vi "Parse Get Topic Rule JSON.vi"(11 "Body":string) -> (3 "Topic Rule":T1)   [LabVIEW 2015, in "NI_AWS_IoT.lvlib"]
uses:
  NI_AWS_IoT.lvlib
  Topic Rule.ctl
  CloudWatch Alarm.ctl
  CloudWatch Metric.ctl
  DynamoDB.ctl
  DynamoDBv2.ctl
  Elasticsearch.ctl
  Firehose.ctl
  Kinesis.ctl
  Lambda.ctl
  Republish.ctl
  S3.ctl
  SNS.ctl
  SQS.ctl
  JSON Parsing/NI_JSON Parsing.lvlib
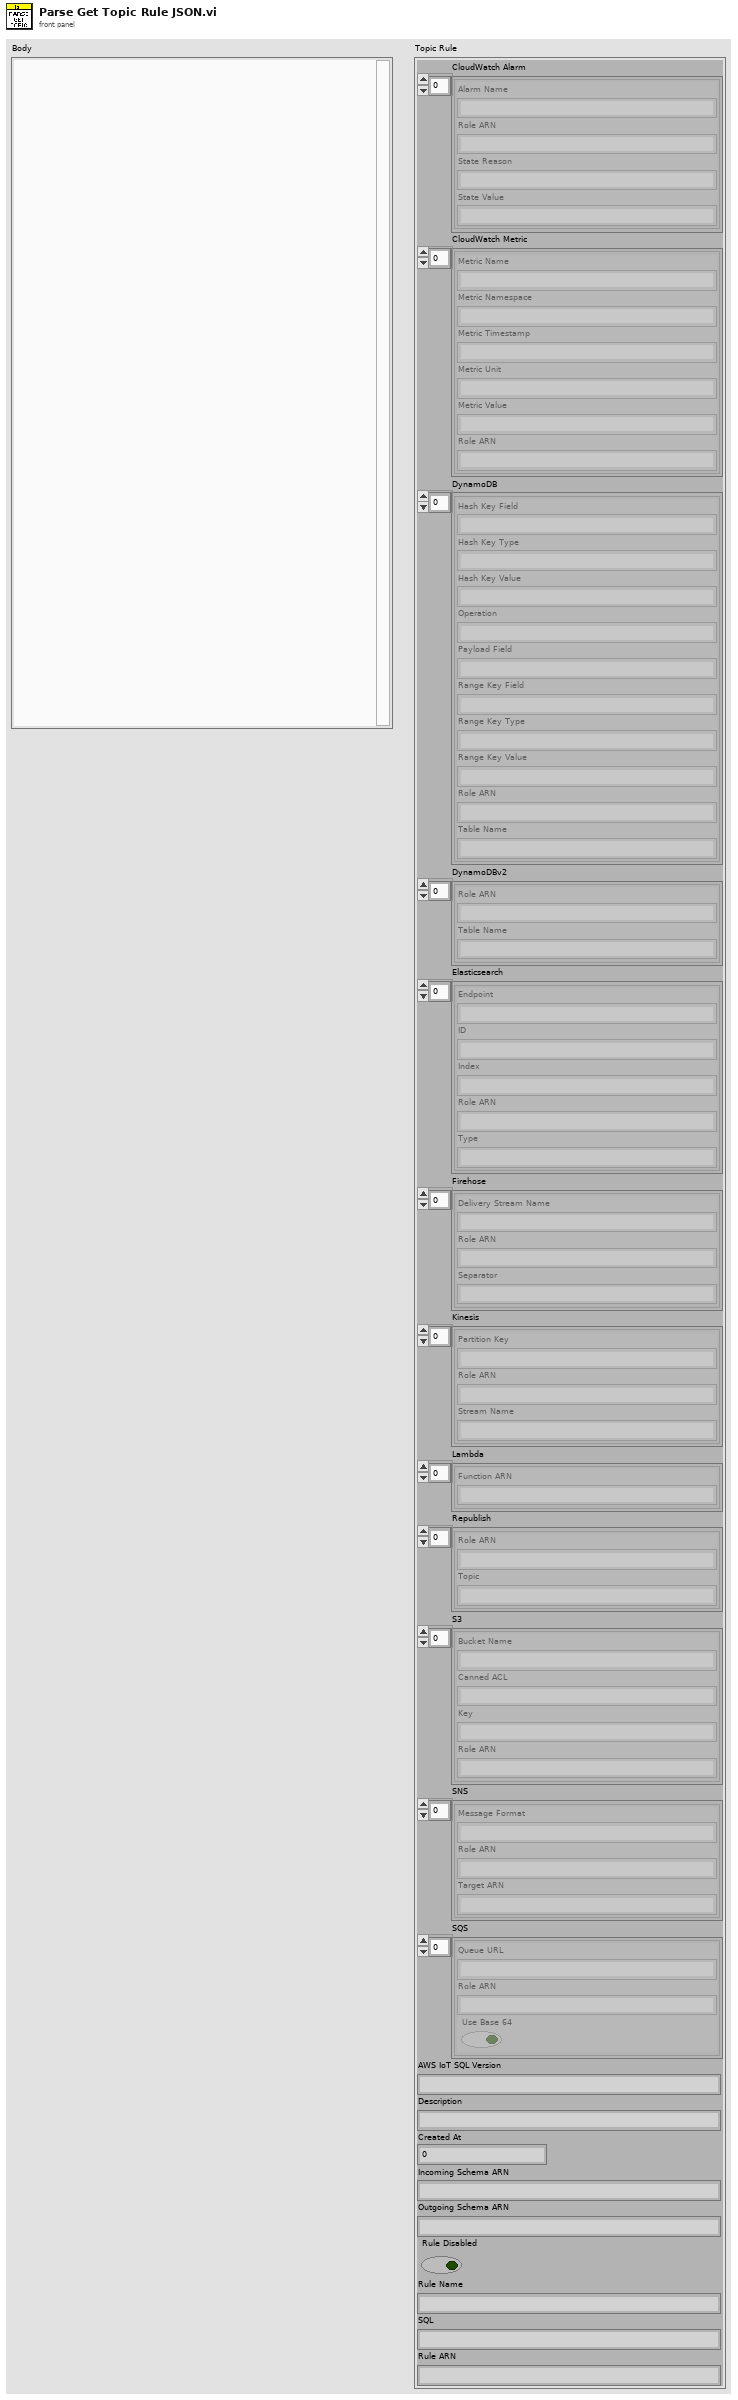
[diagram p1: front panel]
types:
  T1 = typedef "NI_AWS_IoT.lvlib/Topic Rule.ctl" = cluster{"CloudWatch Alarm":T2[], "CloudWatch Metric":T3[], "DynamoDB":T4[], "DynamoDBv2":T5[], "Elasticsearch":T6[], "Firehose":T7[], "Kinesis":T8[], "Lambda":T9[], "Republish":T10[], "S3":T11[], "SNS":T12[], "SQS":T13[], "AWS IoT SQL Version":string, "Description":string, "Created At":u64, "Incoming Schema ARN":string, "Outgoing Schema ARN":string, "Rule Disabled":bool, "Rule Name":string, "SQL":string, "Rule ARN":string}
  T2 = typedef "NI_AWS_IoT.lvlib/CloudWatch Alarm.ctl" = cluster{"Alarm Name":string, "Role ARN":string, "State Reason":string, "State Value":string}
  T3 = typedef "NI_AWS_IoT.lvlib/CloudWatch Metric.ctl" = cluster{"Metric Name":string, "Metric Namespace":string, "Metric Timestamp":string, "Metric Unit":string, "Metric Value":string, "Role ARN":string}
  T4 = typedef "NI_AWS_IoT.lvlib/DynamoDB.ctl" = cluster{"Hash Key Field":string, "Hash Key Type":string, "Hash Key Value":string, "Operation":string, "Payload Field":string, "Range Key Field":string, "Range Key Type":string, "Range Key Value":string, "Role ARN":string, "Table Name":string}
  T5 = typedef "NI_AWS_IoT.lvlib/DynamoDBv2.ctl" = cluster{"Role ARN":string, "Table Name":string}
  T6 = typedef "NI_AWS_IoT.lvlib/Elasticsearch.ctl" = cluster{"Endpoint":string, "ID":string, "Index":string, "Role ARN":string, "Type":string}
  T7 = typedef "NI_AWS_IoT.lvlib/Firehose.ctl" = cluster{"Delivery Stream Name":string, "Role ARN":string, "Separator":string}
  T8 = typedef "NI_AWS_IoT.lvlib/Kinesis.ctl" = cluster{"Partition Key":string, "Role ARN":string, "Stream Name":string}
  T9 = typedef "NI_AWS_IoT.lvlib/Lambda.ctl" = cluster{"Function ARN":string}
  T10 = typedef "NI_AWS_IoT.lvlib/Republish.ctl" = cluster{"Role ARN":string, "Topic":string}
  T11 = typedef "NI_AWS_IoT.lvlib/S3.ctl" = cluster{"Bucket Name":string, "Canned ACL":string, "Key":string, "Role ARN":string}
  T12 = typedef "NI_AWS_IoT.lvlib/SNS.ctl" = cluster{"Message Format":string, "Role ARN":string, "Target ARN":string}
  T13 = typedef "NI_AWS_IoT.lvlib/SQS.ctl" = cluster{"Queue URL":string, "Role ARN":string, "Use Base 64":bool}
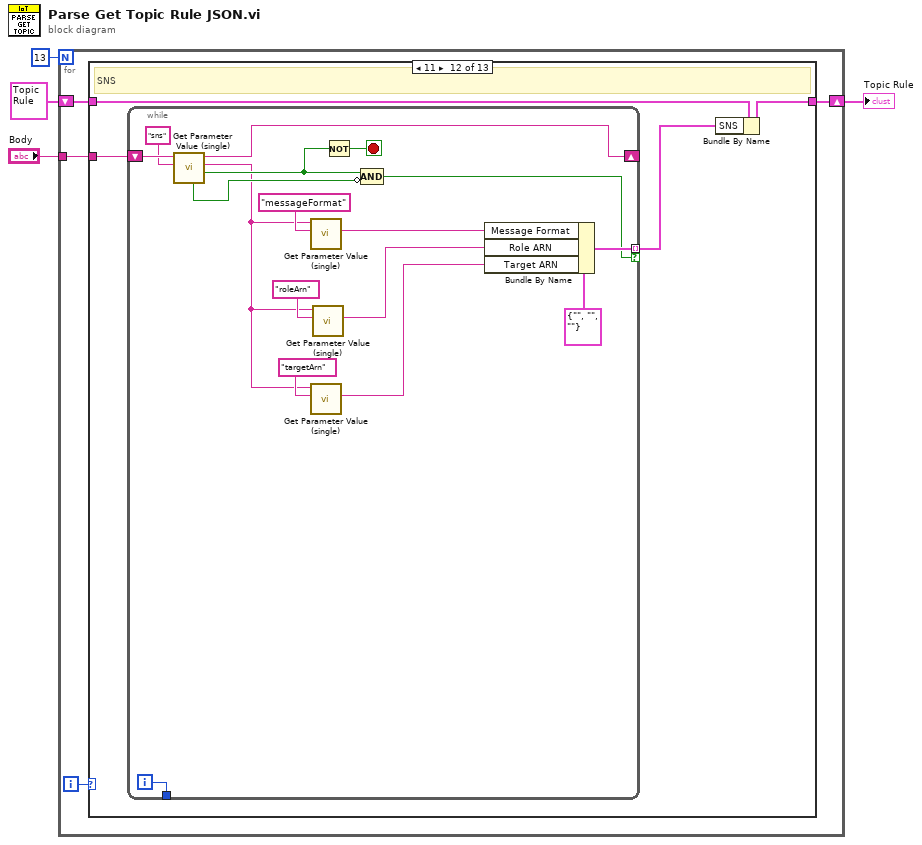
[diagram p0: block diagram]
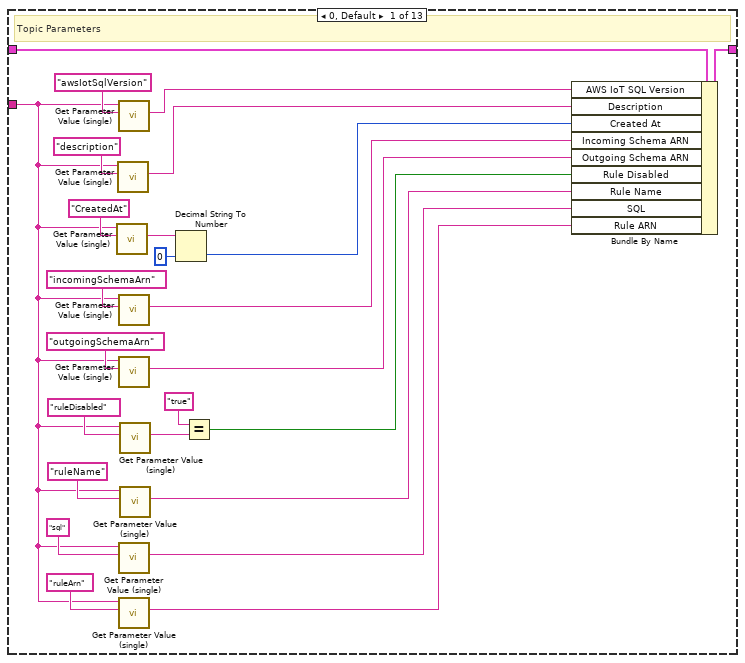
[diagram p2: hidden frame]
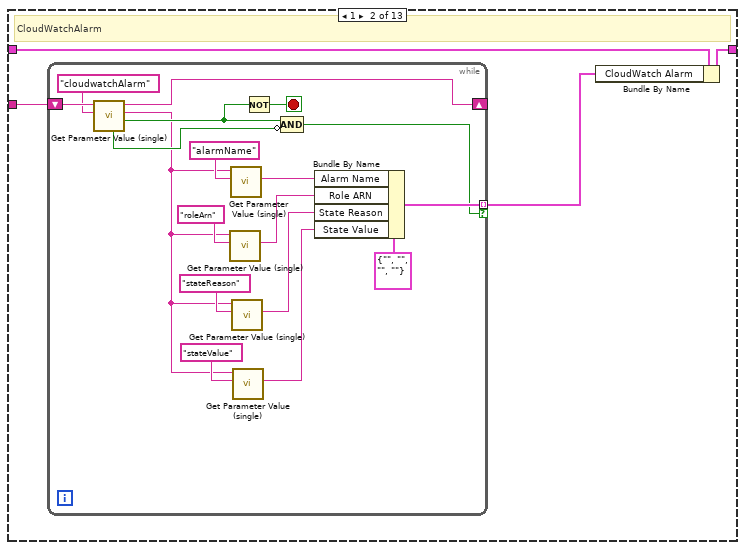
[diagram p3: hidden frame]
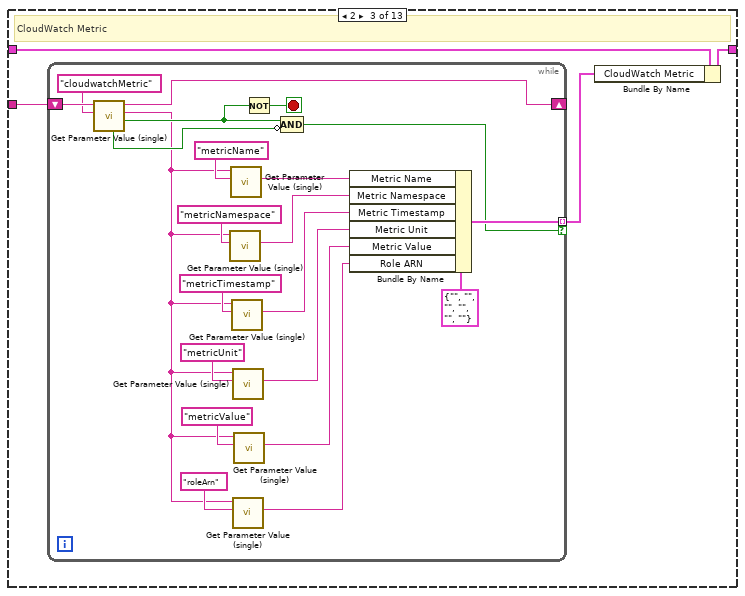
[diagram p4: hidden frame]
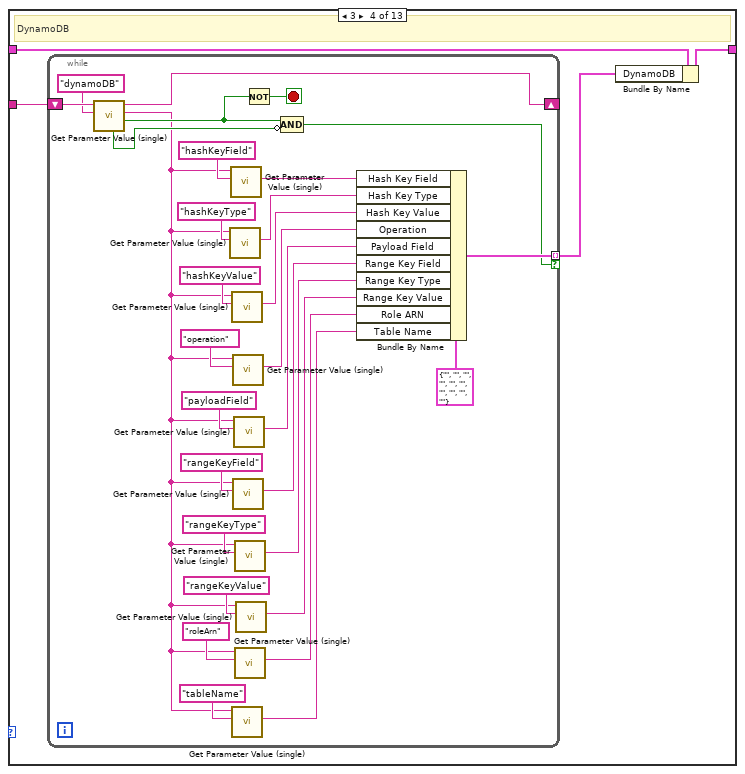
[diagram p5: hidden frame]
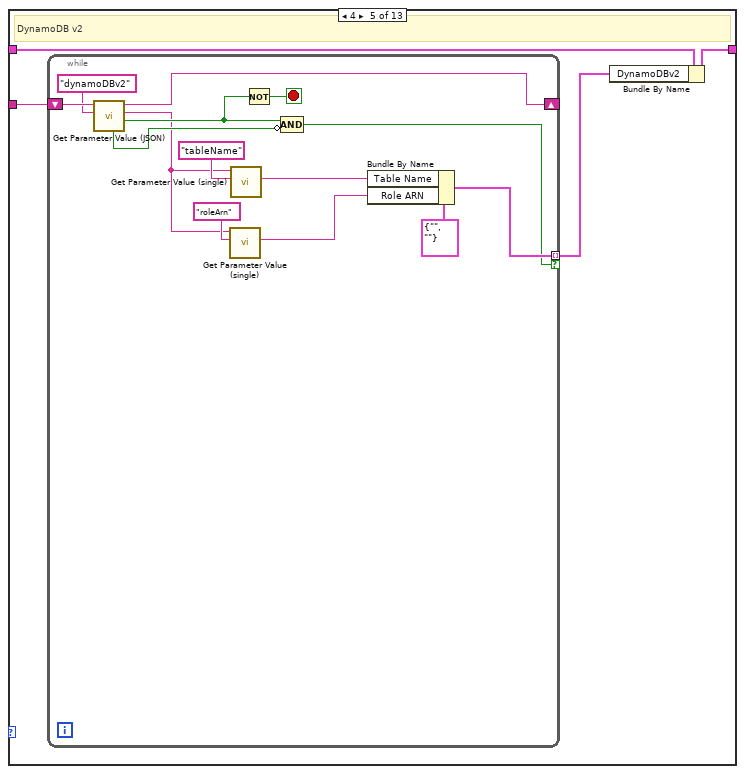
[diagram p6: hidden frame]
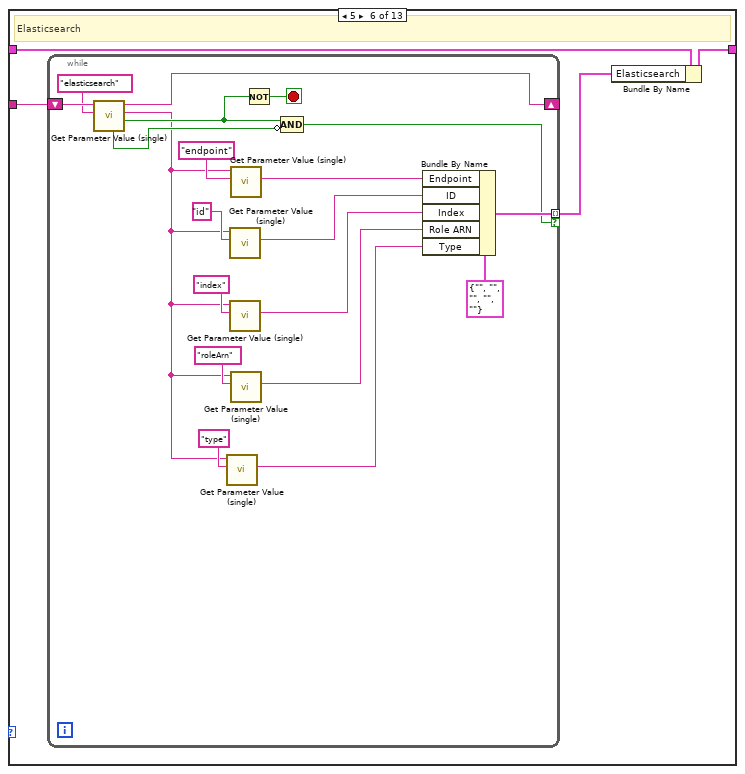
[diagram p7: hidden frame]
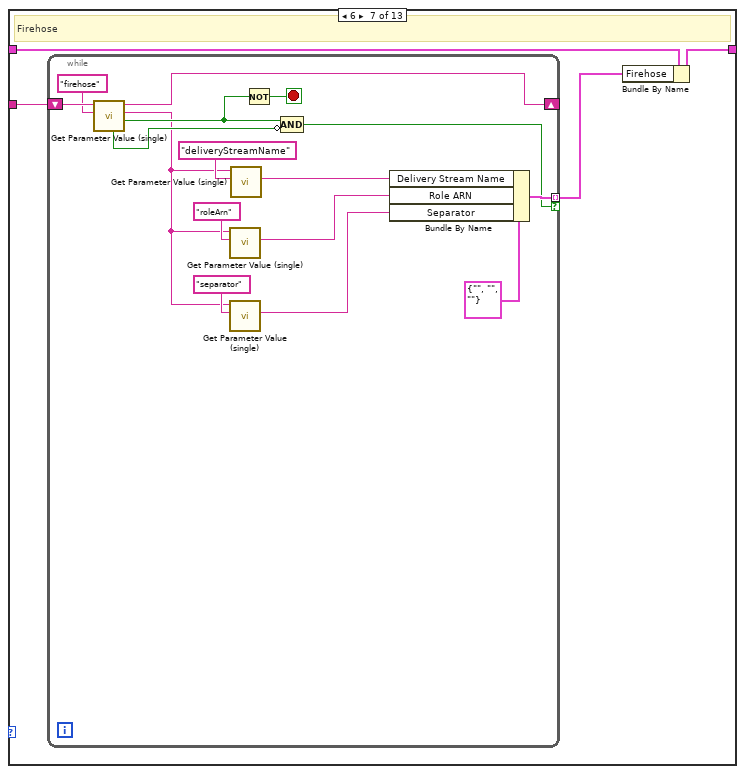
[diagram p8: hidden frame]
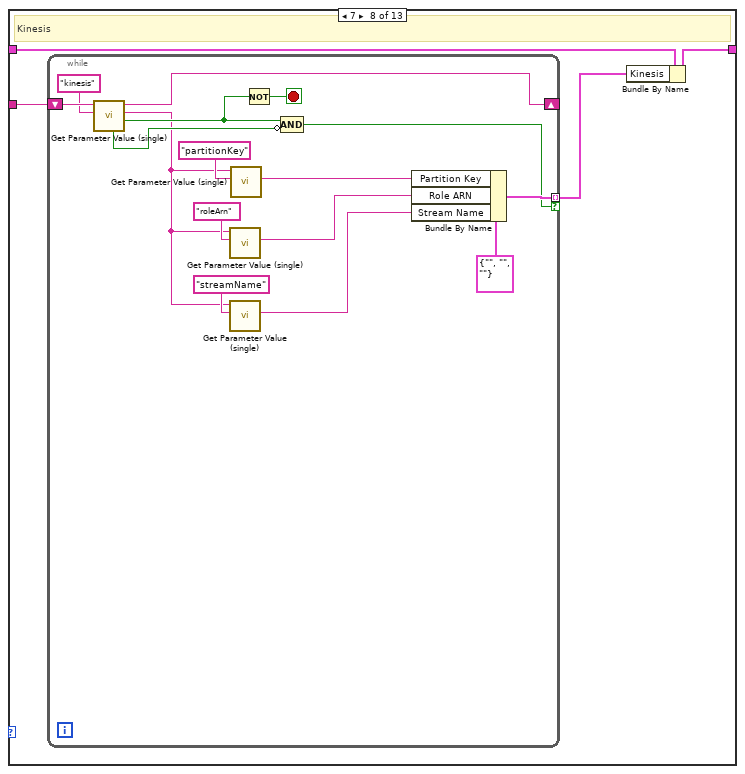
[diagram p9: hidden frame]
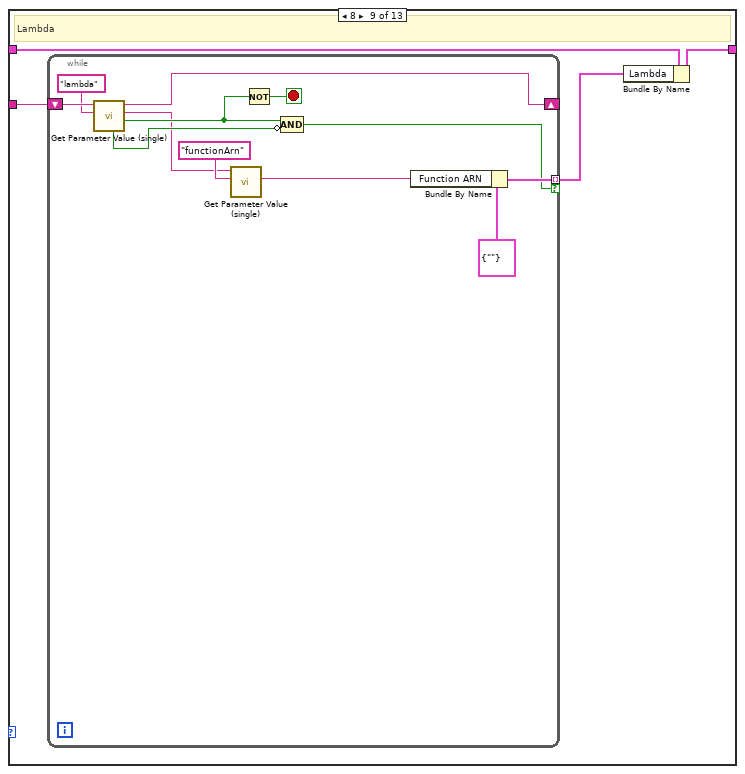
[diagram p10: hidden frame]
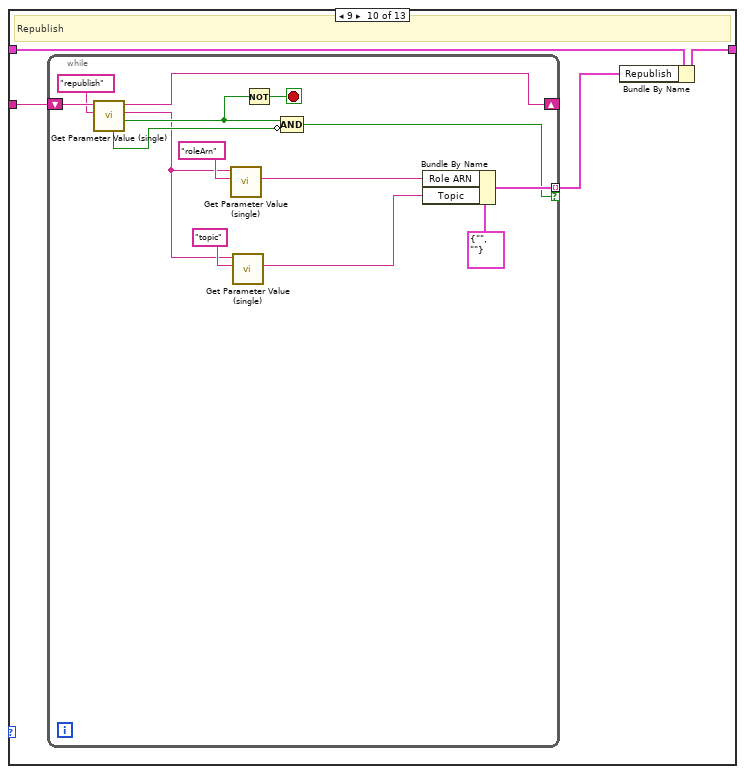
[diagram p11: hidden frame]
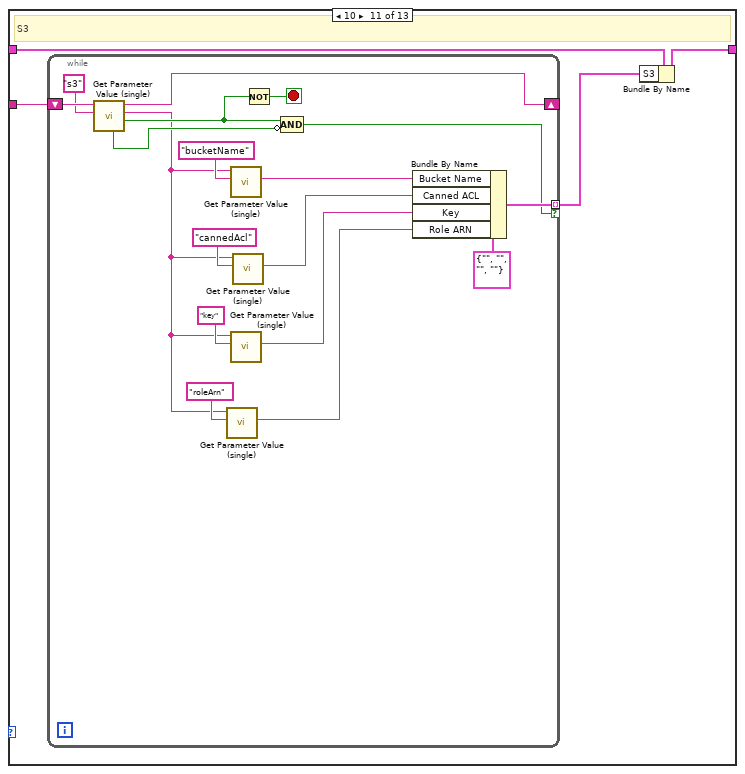
[diagram p12: hidden frame]
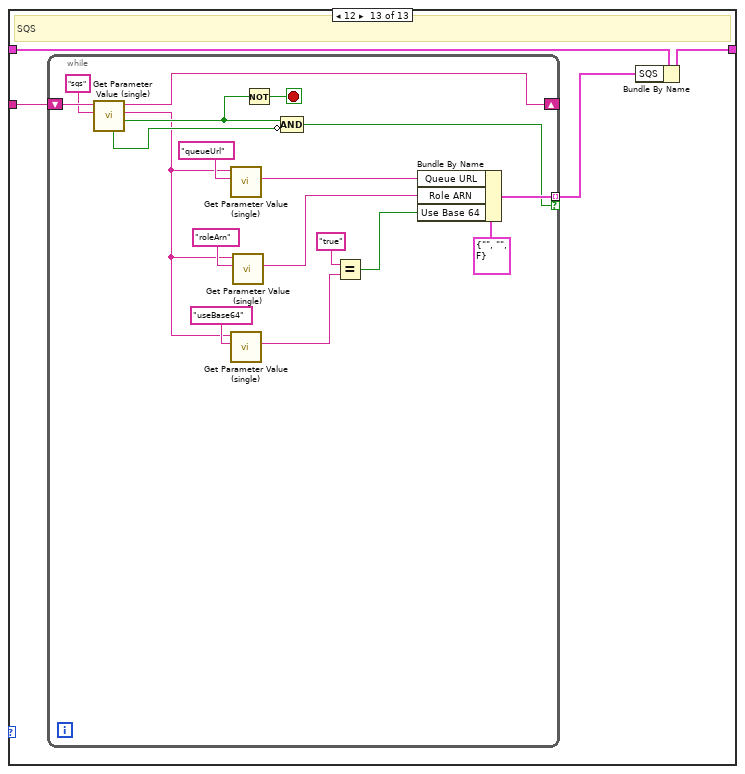
[diagram p13: hidden frame]
diagram:
  n1 = for {
    N: 13 -> [_]
    tunnel: "Body" -> [w5]
    shift-right: [w6] -> w2
    shift-left: T1 {"CloudWatch Alarm"=[], "CloudWatch Metric"=[], "DynamoDB"=[], "DynamoDBv2"=[], "Elasticsearch"=[], "Firehose"=[], "Kinesis"=[], "Lambda"=[], "Republish"=[], "S3"=[], "SNS"=[], "SQS"=[], "AWS IoT SQL Version"="", "Description"="", "Created At"=0, "Incoming Schema ARN"="", "Outgoing Schema ARN"="", "Rule Disabled"=FALSE, "Rule Name"="", "SQL"="", "Rule ARN"=""} ("Topic Rule") -> [w7]
    i -> [w8]
    n2 = case shown="11" w8 {
      tunnel: w7 -> [w33 w37 w59 w85 w119 w137 w161 w181 w201 w217 w235 w257 w278]
      tunnel: [w32 w36 w58 w84 w118 w136 w160 w180 w200 w216 w234 w256 w277] -> w6
      tunnel: w5 -> [w10 w35 w57 w83 w117 w135 w159 w179 w199 w215 w233 w255 w276]
      frame 0, Default {
        # "Topic Parameters"
        n3 = call "Get Parameter Value (single).vi"("Parameter Name"="CreatedAt", "JSON"=w10) -> ("Parameter Value"=w26:string)  [unwired: 6 in, 3 out]
        n4 = call "Get Parameter Value (single).vi"("Parameter Name"="description", "JSON"=w10) -> ("Parameter Value"=w28:string)  [unwired: 6 in, 3 out]
        n5 = call "Get Parameter Value (single).vi"("Parameter Name"="awsIotSqlVersion", "JSON"=w10) -> ("Parameter Value"=w30:string)  [unwired: 6 in, 3 out]
        n6 = call "Get Parameter Value (single).vi"("Parameter Name"="incomingSchemaArn", "JSON"=w10) -> ("Parameter Value"=w22:string)  [unwired: 6 in, 3 out]
        n7 = call "Get Parameter Value (single).vi"("Parameter Name"="outgoingSchemaArn", "JSON"=w10) -> ("Parameter Value"=w20:string)  [unwired: 6 in, 3 out]
        n8 = call "Get Parameter Value (single).vi"("Parameter Name"="sql", "JSON"=w10) -> ("Parameter Value"=w12:string)  [unwired: 6 in, 3 out]
        n9 = call "Get Parameter Value (single).vi"("Parameter Name"="ruleArn", "JSON"=w10) -> ("Parameter Value"=w9:string)  [unwired: 6 in, 3 out]
        n10 = call "Get Parameter Value (single).vi"("Parameter Name"="ruleDisabled", "JSON"=w10) -> ("Parameter Value"=w18:string)  [unwired: 6 in, 3 out]
        n11 = call "Get Parameter Value (single).vi"("Parameter Name"="ruleName", "JSON"=w10) -> ("Parameter Value"=w14:string)  [unwired: 6 in, 3 out]
        n12 = Decimal String To Number(string=w26, default (0L)=u64 0 ("default (0 I32)")) -> (number=w24:u64)  [unwired: 1 in, 1 out]
        n13 = Equal?(x="true", y=w18) -> (x = y?=w16:bool)
        n14 = Bundle By Name(cluster=w33, "AWS IoT SQL Version"=w30, "Description"=w28, "Created At"=w24, "Incoming Schema ARN"=w22, "Outgoing Schema ARN"=w20, "Rule Disabled"=w16, "Rule Name"=w14, "SQL"=w12, "Rule ARN"=w9) -> (w32:T1)
      }
      frame 1 {
        # "CloudWatchAlarm"
        n15 = while {
          shift-right: [w38] -> _
          shift-left: w35 -> [w53]
          tunnel: [w54] -> w34 mode=indexing if=w49
          stop <- w50 stop-if-true
          n16 = call "Get Parameter Value (single).vi"("Parameter Name"="cloudwatchAlarm", "JSON"=w53) -> ("Found"=w51:bool, "Parameter Value"=w39:string, "Remaining JSON"=w38:string, "Null"=w40:bool)  [unwired: 6 in]
          n17 = call "Get Parameter Value (single).vi"("Parameter Name"="roleArn", "JSON"=w39) -> ("Parameter Value"=w43:string)  [unwired: 6 in, 3 out]
          n18 = call "Get Parameter Value (single).vi"("Parameter Name"="alarmName", "JSON"=w39) -> ("Parameter Value"=w44:string)  [unwired: 6 in, 3 out]
          n19 = call "Get Parameter Value (single).vi"("Parameter Name"="stateReason", "JSON"=w39) -> ("Parameter Value"=w42:string)  [unwired: 6 in, 3 out]
          n20 = call "Get Parameter Value (single).vi"("Parameter Name"="stateValue", "JSON"=w39) -> ("Parameter Value"=w41:string)  [unwired: 6 in, 3 out]
          n21 = Not(x=w51) -> (.not. x?=w50:bool)
          n22 = Compound Arithmetic op=AND(w51, invert w40) -> (w49:bool)
          n23 = Bundle By Name(cluster=T2 {"Alarm Name"="", "Role ARN"="", "State Reason"="", "State Value"=""} ("CloudWatch Alarm"), "Alarm Name"=w44, "Role ARN"=w43, "State Reason"=w42, "State Value"=w41) -> (w54:T2)
        }
        n24 = Bundle By Name(cluster=w37, "CloudWatch Alarm"=w34) -> (w36:T1)
      }
      frame 2 {
        # "CloudWatch Metric"
        n25 = while {
          shift-right: [w60] -> _
          shift-left: w57 -> [w80]
          tunnel: [w81] -> w56 mode=indexing if=w76
          stop <- w77 stop-if-true
          n26 = call "Get Parameter Value (single).vi"("Parameter Name"="cloudwatchMetric", "JSON"=w80) -> ("Found"=w78:bool, "Parameter Value"=w61:string, "Remaining JSON"=w60:string, "Null"=w62:bool)  [unwired: 6 in]
          n27 = call "Get Parameter Value (single).vi"("Parameter Name"="metricNamespace", "JSON"=w61) -> ("Parameter Value"=w70:string)  [unwired: 6 in, 3 out]
          n28 = call "Get Parameter Value (single).vi"("Parameter Name"="metricName", "JSON"=w61) -> ("Parameter Value"=w71:string)  [unwired: 6 in, 3 out]
          n29 = call "Get Parameter Value (single).vi"("Parameter Name"="metricTimestamp", "JSON"=w61) -> ("Parameter Value"=w69:string)  [unwired: 6 in, 3 out]
          n30 = call "Get Parameter Value (single).vi"("Parameter Name"="metricUnit", "JSON"=w61) -> ("Parameter Value"=w68:string)  [unwired: 6 in, 3 out]
          n31 = call "Get Parameter Value (single).vi"("Parameter Name"="roleArn", "JSON"=w61) -> ("Parameter Value"=w63:string)  [unwired: 6 in, 3 out]
          n32 = call "Get Parameter Value (single).vi"("Parameter Name"="metricValue", "JSON"=w61) -> ("Parameter Value"=w65:string)  [unwired: 6 in, 3 out]
          n33 = Not(x=w78) -> (.not. x?=w77:bool)
          n34 = Compound Arithmetic op=AND(w78, invert w62) -> (w76:bool)
          n35 = Bundle By Name(cluster=T3 {"Metric Name"="", "Metric Namespace"="", "Metric Timestamp"="", "Metric Unit"="", "Metric Value"="", "Role ARN"=""} ("CloudWatch Metric"), "Metric Name"=w71, "Metric Namespace"=w70, "Metric Timestamp"=w69, "Metric Unit"=w68, "Metric Value"=w65, "Role ARN"=w63) -> (w81:T3)
        }
        n36 = Bundle By Name(cluster=w59, "CloudWatch Metric"=w56) -> (w58:T1)
      }
      frame 3 {
        # "DynamoDB"
        n37 = while {
          shift-right: [w86] -> _
          shift-left: w83 -> [w114]
          tunnel: [w115] -> w82 mode=indexing if=w110
          stop <- w111 stop-if-true
          n38 = call "Get Parameter Value (single).vi"("Parameter Name"="dynamoDB", "JSON"=w114) -> ("Found"=w112:bool, "Parameter Value"=w87:string, "Remaining JSON"=w86:string, "Null"=w88:bool)  [unwired: 6 in]
          n39 = call "Get Parameter Value (single).vi"("Parameter Name"="hashKeyType", "JSON"=w87) -> ("Parameter Value"=w104:string)  [unwired: 6 in, 3 out]
          n40 = call "Get Parameter Value (single).vi"("Parameter Name"="hashKeyField", "JSON"=w87) -> ("Parameter Value"=w105:string)  [unwired: 6 in, 3 out]
          n41 = call "Get Parameter Value (single).vi"("Parameter Name"="hashKeyValue", "JSON"=w87) -> ("Parameter Value"=w103:string)  [unwired: 6 in, 3 out]
          n42 = call "Get Parameter Value (single).vi"("Parameter Name"="tableName", "JSON"=w87) -> ("Parameter Value"=w89:string)  [unwired: 6 in, 3 out]
          n43 = call "Get Parameter Value (single).vi"("Parameter Name"="operation", "JSON"=w87) -> ("Parameter Value"=w102:string)  [unwired: 6 in, 3 out]
          n44 = call "Get Parameter Value (single).vi"("Parameter Name"="rangeKeyField", "JSON"=w87) -> ("Parameter Value"=w98:string)  [unwired: 6 in, 3 out]
          n45 = call "Get Parameter Value (single).vi"("Parameter Name"="payloadField", "JSON"=w87) -> ("Parameter Value"=w100:string)  [unwired: 6 in, 3 out]
          n46 = call "Get Parameter Value (single).vi"("Parameter Name"="rangeKeyType", "JSON"=w87) -> ("Parameter Value"=w95:string)  [unwired: 6 in, 3 out]
          n47 = call "Get Parameter Value (single).vi"("Parameter Name"="roleArn", "JSON"=w87) -> ("Parameter Value"=w91:string)  [unwired: 6 in, 3 out]
          n48 = call "Get Parameter Value (single).vi"("Parameter Name"="rangeKeyValue", "JSON"=w87) -> ("Parameter Value"=w93:string)  [unwired: 6 in, 3 out]
          n49 = Not(x=w112) -> (.not. x?=w111:bool)
          n50 = Compound Arithmetic op=AND(w112, invert w88) -> (w110:bool)
          n51 = Bundle By Name(cluster=T4 {"Hash Key Field"="", "Hash Key Type"="", "Hash Key Value"="", "Operation"="", "Payload Field"="", "Range Key Field"="", "Range Key Type"="", "Range Key Value"="", "Role ARN"="", "Table Name"=""} ("DynamoDB"), "Hash Key Field"=w105, "Hash Key Type"=w104, "Hash Key Value"=w103, "Operation"=w102, "Payload Field"=w100, "Range Key Field"=w98, "Range Key Type"=w95, "Range Key Value"=w93, "Role ARN"=w91, "Table Name"=w89) -> (w115:T4)
        }
        n52 = Bundle By Name(cluster=w85, "DynamoDB"=w82) -> (w84:T1)
      }
      frame 4 {
        # "DynamoDB v2"
        n53 = while {
          shift-right: [w122] -> _
          shift-left: w117 -> [w121]
          tunnel: [w133] -> w116 mode=indexing if=w130
          stop <- w131 stop-if-true
          n54 = call "Get Parameter Value (JSON).vi"("Parameter Name"="dynamoDBv2", "JSON"=w121) -> ("Found"=w132:bool, "Parameter Value"=w123:string, "Remaining JSON"=w122:string, "Null"=w125:bool)  [unwired: 6 in]
          n55 = call "Get Parameter Value (single).vi"("Parameter Name"="roleArn", "JSON"=w123) -> ("Parameter Value"=w126:string)  [unwired: 6 in, 3 out]
          n56 = call "Get Parameter Value (single).vi"("Parameter Name"="tableName", "JSON"=w123) -> ("Parameter Value"=w127:string)  [unwired: 6 in, 3 out]
          n57 = Not(x=w132) -> (.not. x?=w131:bool)
          n58 = Compound Arithmetic op=AND(w132, invert w125) -> (w130:bool)
          n59 = Bundle By Name(cluster=T5 {"Role ARN"="", "Table Name"=""} ("DynamoDBv2"), "Table Name"=w127, "Role ARN"=w126) -> (w133:T5)
        }
        n60 = Bundle By Name(cluster=w119, "DynamoDBv2"=w116) -> (w118:T1)
      }
      frame 5 {
        # "Elasticsearch"
        n61 = while {
          shift-right: [w138] -> _
          shift-left: w135 -> [w156]
          tunnel: [w157] -> w134 mode=indexing if=w152
          stop <- w153 stop-if-true
          n62 = call "Get Parameter Value (single).vi"("Parameter Name"="elasticsearch", "JSON"=w156) -> ("Found"=w154:bool, "Parameter Value"=w139:string, "Remaining JSON"=w138:string, "Null"=w147:bool)  [unwired: 6 in]
          n63 = call "Get Parameter Value (single).vi"("Parameter Name"="type", "JSON"=w139) -> ("Parameter Value"=w140:string)  [unwired: 6 in, 3 out]
          n64 = call "Get Parameter Value (single).vi"("Parameter Name"="id", "JSON"=w139) -> ("Parameter Value"=w148:string)  [unwired: 6 in, 3 out]
          n65 = call "Get Parameter Value (single).vi"("Parameter Name"="index", "JSON"=w139) -> ("Parameter Value"=w142:string)  [unwired: 6 in, 3 out]
          n66 = call "Get Parameter Value (single).vi"("Parameter Name"="endpoint", "JSON"=w139) -> ("Parameter Value"=w149:string)  [unwired: 6 in, 3 out]
          n67 = call "Get Parameter Value (single).vi"("Parameter Name"="roleArn", "JSON"=w139) -> ("Parameter Value"=w141:string)  [unwired: 6 in, 3 out]
          n68 = Not(x=w154) -> (.not. x?=w153:bool)
          n69 = Compound Arithmetic op=AND(w154, invert w147) -> (w152:bool)
          n70 = Bundle By Name(cluster=T6 {"Endpoint"="", "ID"="", "Index"="", "Role ARN"="", "Type"=""} ("Elasticsearch"), "Endpoint"=w149, "ID"=w148, "Index"=w142, "Role ARN"=w141, "Type"=w140) -> (w157:T6)
        }
        n71 = Bundle By Name(cluster=w137, "Elasticsearch"=w134) -> (w136:T1)
      }
      frame 6 {
        # "Firehose"
        n72 = while {
          shift-right: [w162] -> _
          shift-left: w159 -> [w176]
          tunnel: [w177] -> w158 mode=indexing if=w172
          stop <- w173 stop-if-true
          n73 = call "Get Parameter Value (single).vi"("Parameter Name"="firehose", "JSON"=w176) -> ("Found"=w174:bool, "Parameter Value"=w163:string, "Remaining JSON"=w162:string, "Null"=w167:bool)  [unwired: 6 in]
          n74 = call "Get Parameter Value (single).vi"("Parameter Name"="roleArn", "JSON"=w163) -> ("Parameter Value"=w168:string)  [unwired: 6 in, 3 out]
          n75 = call "Get Parameter Value (single).vi"("Parameter Name"="separator", "JSON"=w163) -> ("Parameter Value"=w165:string)  [unwired: 6 in, 3 out]
          n76 = call "Get Parameter Value (single).vi"("Parameter Name"="deliveryStreamName", "JSON"=w163) -> ("Parameter Value"=w169:string)  [unwired: 6 in, 3 out]
          n77 = Not(x=w174) -> (.not. x?=w173:bool)
          n78 = Compound Arithmetic op=AND(w174, invert w167) -> (w172:bool)
          n79 = Bundle By Name(cluster=T7 {"Delivery Stream Name"="", "Role ARN"="", "Separator"=""} ("Firehose"), "Delivery Stream Name"=w169, "Role ARN"=w168, "Separator"=w165) -> (w177:T7)
        }
        n80 = Bundle By Name(cluster=w161, "Firehose"=w158) -> (w160:T1)
      }
      frame 7 {
        # "Kinesis"
        n81 = while {
          shift-right: [w182] -> _
          shift-left: w179 -> [w196]
          tunnel: [w197] -> w178 mode=indexing if=w192
          stop <- w193 stop-if-true
          n82 = call "Get Parameter Value (single).vi"("Parameter Name"="kinesis", "JSON"=w196) -> ("Found"=w194:bool, "Parameter Value"=w183:string, "Remaining JSON"=w182:string, "Null"=w187:bool)  [unwired: 6 in]
          n83 = call "Get Parameter Value (single).vi"("Parameter Name"="roleArn", "JSON"=w183) -> ("Parameter Value"=w188:string)  [unwired: 6 in, 3 out]
          n84 = call "Get Parameter Value (single).vi"("Parameter Name"="streamName", "JSON"=w183) -> ("Parameter Value"=w185:string)  [unwired: 6 in, 3 out]
          n85 = call "Get Parameter Value (single).vi"("Parameter Name"="partitionKey", "JSON"=w183) -> ("Parameter Value"=w189:string)  [unwired: 6 in, 3 out]
          n86 = Not(x=w194) -> (.not. x?=w193:bool)
          n87 = Compound Arithmetic op=AND(w194, invert w187) -> (w192:bool)
          n88 = Bundle By Name(cluster=T8 {"Partition Key"="", "Role ARN"="", "Stream Name"=""} ("Kinesis"), "Partition Key"=w189, "Role ARN"=w188, "Stream Name"=w185) -> (w197:T8)
        }
        n89 = Bundle By Name(cluster=w181, "Kinesis"=w178) -> (w180:T1)
      }
      frame 8 {
        # "Lambda"
        n90 = while {
          shift-right: [w202] -> _
          shift-left: w199 -> [w212]
          tunnel: [w213] -> w198 mode=indexing if=w208
          stop <- w209 stop-if-true
          n91 = call "Get Parameter Value (single).vi"("Parameter Name"="lambda", "JSON"=w212) -> ("Found"=w210:bool, "Parameter Value"=w203:string, "Remaining JSON"=w202:string, "Null"=w205:bool)  [unwired: 6 in]
          n92 = call "Get Parameter Value (single).vi"("Parameter Name"="functionArn", "JSON"=w203) -> ("Parameter Value"=w206:string)  [unwired: 6 in, 3 out]
          n93 = Not(x=w210) -> (.not. x?=w209:bool)
          n94 = Compound Arithmetic op=AND(w210, invert w205) -> (w208:bool)
          n95 = Bundle By Name(cluster=T9 {"Function ARN"=""} ("Lambda"), "Function ARN"=w206) -> (w213:T9)
        }
        n96 = Bundle By Name(cluster=w201, "Lambda"=w198) -> (w200:T1)
      }
      frame 9 {
        # "Republish"
        n97 = while {
          shift-right: [w218] -> _
          shift-left: w215 -> [w230]
          tunnel: [w231] -> w214 mode=indexing if=w226
          stop <- w227 stop-if-true
          n98 = call "Get Parameter Value (single).vi"("Parameter Name"="republish", "JSON"=w230) -> ("Found"=w228:bool, "Parameter Value"=w219:string, "Remaining JSON"=w218:string, "Null"=w223:bool)  [unwired: 6 in]
          n99 = call "Get Parameter Value (single).vi"("Parameter Name"="roleArn", "JSON"=w219) -> ("Parameter Value"=w224:string)  [unwired: 6 in, 3 out]
          n100 = call "Get Parameter Value (single).vi"("Parameter Name"="topic", "JSON"=w219) -> ("Parameter Value"=w220:string)  [unwired: 6 in, 3 out]
          n101 = Not(x=w228) -> (.not. x?=w227:bool)
          n102 = Compound Arithmetic op=AND(w228, invert w223) -> (w226:bool)
          n103 = Bundle By Name(cluster=T10 {"Role ARN"="", "Topic"=""} ("Republish"), "Role ARN"=w224, "Topic"=w220) -> (w231:T10)
        }
        n104 = Bundle By Name(cluster=w217, "Republish"=w214) -> (w216:T1)
      }
      frame 10 {
        # "S3"
        n105 = while {
          shift-right: [w236] -> _
          shift-left: w233 -> [w252]
          tunnel: [w253] -> w232 mode=indexing if=w248
          stop <- w249 stop-if-true
          n106 = call "Get Parameter Value (single).vi"("Parameter Name"="s3", "JSON"=w252) -> ("Found"=w250:bool, "Parameter Value"=w237:string, "Remaining JSON"=w236:string, "Null"=w245:bool)  [unwired: 6 in]
          n107 = call "Get Parameter Value (single).vi"("Parameter Name"="roleArn", "JSON"=w237) -> ("Parameter Value"=w238:string)  [unwired: 6 in, 3 out]
          n108 = call "Get Parameter Value (single).vi"("Parameter Name"="bucketName", "JSON"=w237) -> ("Parameter Value"=w246:string)  [unwired: 6 in, 3 out]
          n109 = call "Get Parameter Value (single).vi"("Parameter Name"="key", "JSON"=w237) -> ("Parameter Value"=w239:string)  [unwired: 6 in, 3 out]
          n110 = call "Get Parameter Value (single).vi"("Parameter Name"="cannedAcl", "JSON"=w237) -> ("Parameter Value"=w243:string)  [unwired: 6 in, 3 out]
          n111 = Not(x=w250) -> (.not. x?=w249:bool)
          n112 = Compound Arithmetic op=AND(w250, invert w245) -> (w248:bool)
          n113 = Bundle By Name(cluster=T11 {"Bucket Name"="", "Canned ACL"="", "Key"="", "Role ARN"=""} ("S3"), "Bucket Name"=w246, "Canned ACL"=w243, "Key"=w239, "Role ARN"=w238) -> (w253:T11)
        }
        n114 = Bundle By Name(cluster=w235, "S3"=w232) -> (w234:T1)
      }
      frame 11 {
        # "SNS"
        n115 = while {
          shift-right: [w258] -> _
          shift-left: w255 -> [w273]
          tunnel: [w274] -> w254 mode=indexing if=w269
          tunnel: [w260] -> _
          i -> [w260]
          stop <- w270 stop-if-true
          n116 = call "Get Parameter Value (single).vi"("Parameter Name"="sns", "JSON"=w273) -> ("Found"=w271:bool, "Parameter Value"=w259:string, "Remaining JSON"=w258:string, "Null"=w266:bool)  [unwired: 6 in]
          n117 = call "Get Parameter Value (single).vi"("Parameter Name"="messageFormat", "JSON"=w259) -> ("Parameter Value"=w267:string)  [unwired: 6 in, 3 out]
          n118 = call "Get Parameter Value (single).vi"("Parameter Name"="targetArn", "JSON"=w259) -> ("Parameter Value"=w262:string)  [unwired: 6 in, 3 out]
          n119 = call "Get Parameter Value (single).vi"("Parameter Name"="roleArn", "JSON"=w259) -> ("Parameter Value"=w264:string)  [unwired: 6 in, 3 out]
          n120 = Not(x=w271) -> (.not. x?=w270:bool)
          n121 = Compound Arithmetic op=AND(w271, invert w266) -> (w269:bool)
          n122 = Bundle By Name(cluster=T12 {"Message Format"="", "Role ARN"="", "Target ARN"=""} ("SNS"), "Message Format"=w267, "Role ARN"=w264, "Target ARN"=w262) -> (w274:T12)
        }
        n123 = Bundle By Name(cluster=w257, "SNS"=w254) -> (w256:T1)
      }
      frame 12 {
        # "SQS"
        n124 = while {
          shift-right: [w279] -> _
          shift-left: w276 -> [w295]
          tunnel: [w296] -> w275 mode=indexing if=w291
          stop <- w292 stop-if-true
          n125 = call "Get Parameter Value (single).vi"("Parameter Name"="sqs", "JSON"=w295) -> ("Found"=w293:bool, "Parameter Value"=w280:string, "Remaining JSON"=w279:string, "Null"=w288:bool)  [unwired: 6 in]
          n126 = call "Get Parameter Value (single).vi"("Parameter Name"="queueUrl", "JSON"=w280) -> ("Parameter Value"=w289:string)  [unwired: 6 in, 3 out]
          n127 = call "Get Parameter Value (single).vi"("Parameter Name"="useBase64", "JSON"=w280) -> ("Parameter Value"=w283:string)  [unwired: 6 in, 3 out]
          n128 = call "Get Parameter Value (single).vi"("Parameter Name"="roleArn", "JSON"=w280) -> ("Parameter Value"=w286:string)  [unwired: 6 in, 3 out]
          n129 = Not(x=w293) -> (.not. x?=w292:bool)
          n130 = Compound Arithmetic op=AND(w293, invert w288) -> (w291:bool)
          n131 = Equal?(x="true", y=w283) -> (x = y?=w281:bool)
          n132 = Bundle By Name(cluster=T13 {"Queue URL"="", "Role ARN"="", "Use Base 64"=FALSE} ("SQS"), "Queue URL"=w289, "Role ARN"=w286, "Use Base 64"=w281) -> (w296:T13)
        }
        n133 = Bundle By Name(cluster=w278, "SQS"=w275) -> (w277:T1)
      }
    }
  }
  "Topic Rule" <- w2
